vi "Start Scan.vi"(8 "error in (no error)":errorcluster, 9 "Scan Settings":T1, 10 "Model in":refnum<class "Model.lvclass">, 11 "State in":refnum<class "State.lvclass">) -> (0 "error out":errorcluster, 2 "Model out":refnum<class "Model.lvclass">, 3 "State out":refnum<class "State.lvclass">)   [LabVIEW 2015, in "State.lvclass"]
uses:
  State.lvclass
  Model/Model/Model.lvclass
  Typedefs/ScanSettings.ctl
  Typedefs/WaveformSettings.ctl
  Typedefs/WaveformTypes.ctl
  Typedefs/FAMT Typedefs.lvlib
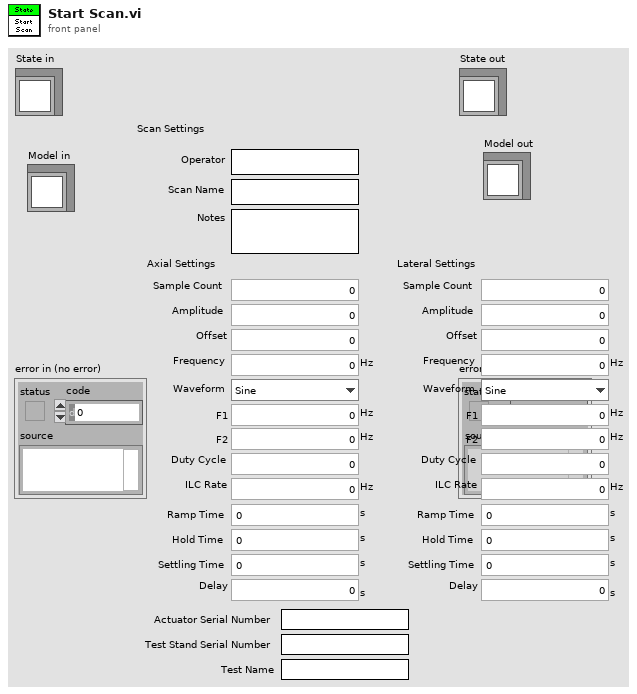
[diagram p1: front panel]
types:
  T1 = typedef "FAMT Typedefs.lvlib/ScanSettings.ctl" = cluster{"Operator":string, "Scan Name":string, "Notes":string, "Axial Settings":T2, "Lateral Settings":T2, "Actuator Serial Number":string, "Test Stand Serial Number":string, "Test Name":string}
  T2 = typedef "FAMT Typedefs.lvlib/WaveformSettings.ctl" = cluster{"Sample Count":u32, "Amplitude":dbl, "Offset":dbl, "Frequency":dbl[unit], "Waveform":T3, "F1":dbl[unit], "F2":dbl[unit], "Duty Cycle":dbl, "ILC Rate":dbl[unit], "Ramp Time":dbl[unit], "Hold Time":dbl[unit], "Settling Time":dbl[unit], "Delay":dbl[unit]}
  T3 = typedef "FAMT Typedefs.lvlib/WaveformTypes.ctl" = enum16{"Sine", "Triangle", "Square", "Sawtooth", "Chirp", "Gaussian", "Trapezoid", "Constant"}
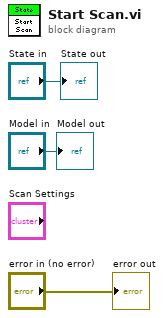
[diagram p0: block diagram]
diagram:
  "error out" <- "error in (no error)"
  "State out" <- "State in"
  "Model out" <- "Model in"
